vi "GDSProject_CreateFolder.vi"(0 "Project Refnum In":refnum<vi>, 1 "Project Item To Create Folder Below(Use MyComputer if not wired)":refnum<vi>, 3 "FolderName":string, 5 "error in (no error)":errorcluster, 7 "FolderScope":T1(array[ring]), 8 "CreateThePhysicalFolderIfPossible(False)":bool, 9 "GuessFolderScope(False)":bool) -> (14 "Project Refnum Out":refnum<vi>, 15 "ItemOut":refnum<vi>, 16 "FolderCreated":bool, 19 "error out":errorcluster)   [LabVIEW 2016]
panel:
  # "E.g. Private/SubPrivate"
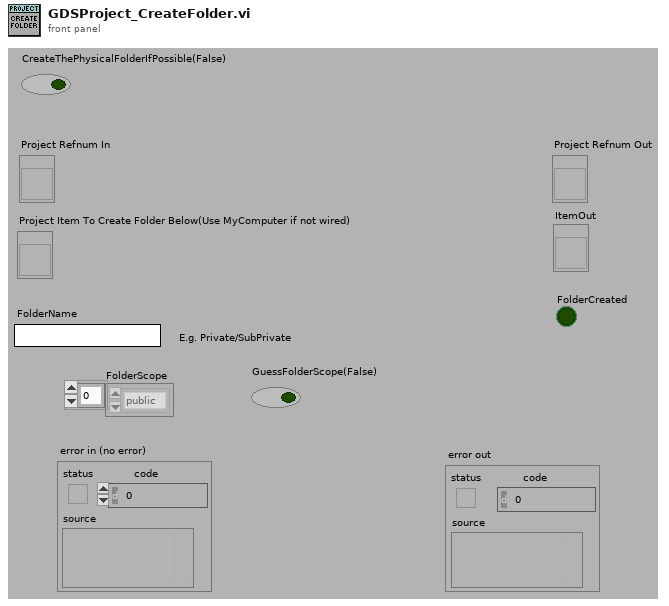
[diagram p1: front panel]
types:
  T1 = enum32{"invalid scope", "public", "private", "protected", "community"}[]
  T2 = enum32{"invalid scope", "public", "private", "protected"}
  T3 = enum32{"invalid scope", "public", "private", "protected", "community"}
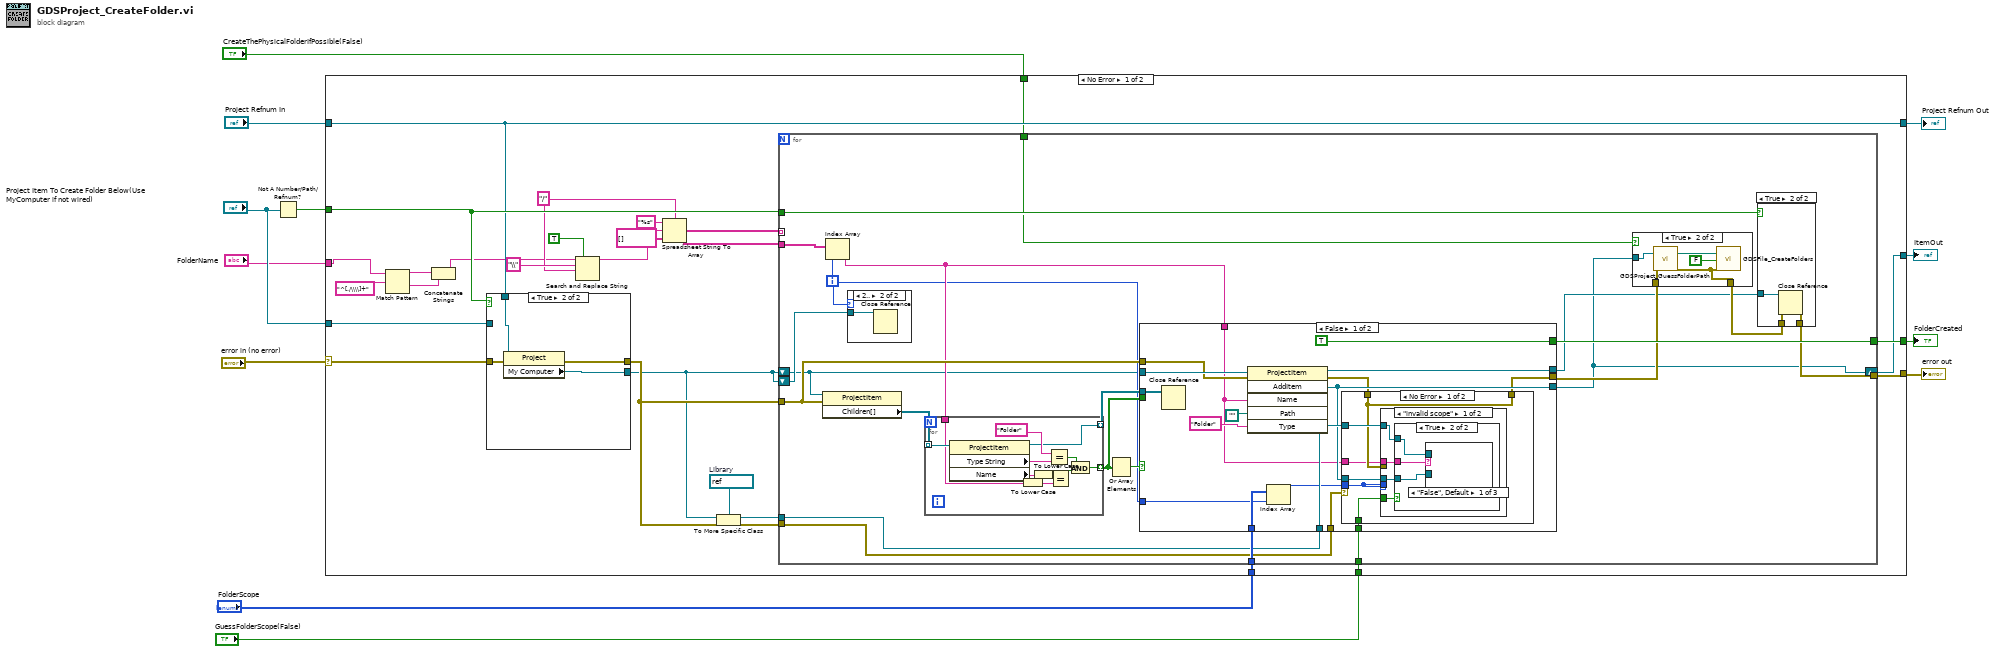
[diagram p0: block diagram]
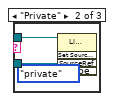
[diagram p5: hidden frame]
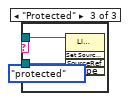
[diagram p6: hidden frame]
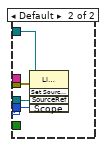
[diagram p7: hidden frame]
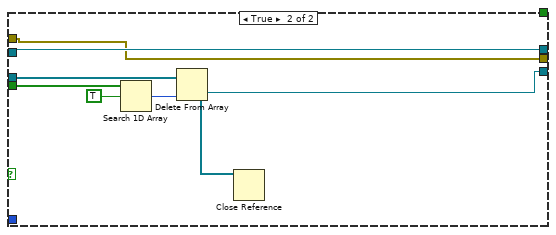
[diagram p9: hidden frame]
diagram:
  n1 = Not A Number/Path/Refnum?(number/path/refnum="Project Item To Create Folder Below(Use MyComputer if not wired)") -> (NaN/Path/Refnum?=w9:bool)
  n2 = case shown="No Error" "error in (no error)" {
    selector: "error in (no error)" -> [w39 w140]
    tunnel: [w33 w140] -> w11
    tunnel: "Project Refnum In" -> [w36 w139]
    tunnel: w9 -> [w37 _]
    tunnel: "Project Item To Create Folder Below(Use MyComputer if not wired)" -> [w38 _]
    tunnel: [w36 w139] -> w7
    tunnel: "FolderName" -> [w14 _]
    tunnel: [w29 _] -> w5
    tunnel: [w35 _] -> w4
    tunnel: "CreateThePhysicalFolderIfPossible(False)" -> [w34 _]
    tunnel: "FolderScope" -> [w28 _]
    tunnel: "GuessFolderScope(False)" -> [w18 _]
    frame No Error {
      w23 = refnum<vi> refnum  # Library
      w26 = "/" ("delimiter (Tab)")
      n3 = Match Pattern(string=w14, regular expression="^[./\\\\]+") -> (before substring=w16:string, after substring=w15:string)  [unwired: 1 in, 2 out]
      n4 = Concatenate Strings(w16, w15) -> (w13:string)
      n5 = case shown="True" w37 {
        tunnel: w36 -> [_ w138]
        tunnel: w39 -> [w133 w137]
        tunnel: [w134 w136] -> w19
        tunnel: w38 -> [w134 _]
        tunnel: [w133 w135] -> w20
        frame False {
        }
        frame True {
          n6 = property class="Project"(reference=w138, error in=w137) -> (error out=w135:errorcluster, "My Computer"=w136:refnum<vi>)  [unwired: 1 out]
        }
      }
      n7 = Search and Replace String(replace all?=TRUE ("replace all? (F)"), input string=w13, search string="\\", replace string=w26) -> (result string=w24:string)  [unwired: 4 in, 3 out]
      n8 = Spreadsheet String To Array(delimiter (Tab)=w26, format string="%s", spreadsheet string=w24, array type (2D Dbl)=string[] []) -> (array=w30:string[])
      n9 = To More Specific Class(target class=w23, reference=w19, error in=w20) -> (specific class reference=w22:refnum<vi>, error out=w21:errorcluster)
      n10 = for {
        tunnel: w37 -> [w61]
        tunnel: w20 -> [w60]
        tunnel: [w55] -> w35
        tunnel: w34 -> [w54]
        tunnel: [w51] -> w33
        tunnel: w30 -> [_] mode=indexing
        tunnel: w30 -> [w49]
        shift-right: [w47] -> w29
        shift-left: w19 -> [w43]
        shift-left: w19 -> [w46]
        tunnel: w28 -> [w45]
        tunnel: w22 -> [w42]
        tunnel: w21 -> [w41]
        tunnel: w18 -> [w40]
        i -> [w44]
        n11 = property class="ProjectItem"(reference=w43, error in=w60) -> ("Children[]"=w59:refnum<vi>[])  [unwired: 2 out]
        n12 = Index Array(array=w49, index=w44) -> (element=w48:string)
        n13 = case shown="2.." w44 {
          tunnel: w46 -> [_ w62]
          frame 0, Default {
          }
          frame 2.. {
            n14 = Close Reference(reference=w62) -> ()  [unwired: 1 in, 1 out]
          }
        }
        n15 = for {
          tunnel: w59 -> [w128] mode=indexing
          tunnel: w48 -> [w124]
          tunnel: [w121] -> w57 mode=indexing
          tunnel: [w120] -> w56 mode=indexing
          n16 = property class="ProjectItem"(reference=w128) -> (reference out=w120:refnum<vi>, "Type String"=w127:string, "Name"=w125:string)  [unwired: 1 in, 1 out]
          n17 = To Lower Case(string=w124) -> (all lower case string=w118:string)
          n18 = To Lower Case(string=w125) -> (all lower case string=w119:string)
          n19 = Equal?(x="Folder", y=w127) -> (x = y?=w123:bool)
          n20 = Equal?(x=w119, y=w118) -> (x = y?=w122:bool)
          n21 = And(x=w123, y=w122) -> (x .and. y?=w121:bool)
        }
        n22 = Or Array Elements(Boolean array=w57) -> (logical OR=w58:bool)
        n23 = case shown="False" w58 {
          tunnel: [w72 w111] -> w53
          tunnel: [w75 w113] -> w47
          tunnel: [w84 w112] -> w50
          tunnel: w43 -> [w82 w112]
          tunnel: w60 -> [w81 w111]
          tunnel: w48 -> [w70 _]
          tunnel: w57 -> [_ w117]
          tunnel: w56 -> [w69 w115]
          tunnel: [TRUE _] -> w55
          tunnel: w45 -> [w79 _]
          tunnel: w44 -> [w78 _]
          tunnel: w41 -> [w77 _]
          tunnel: w42 -> [w76 _]
          tunnel: w40 -> [w71 _]
          frame False {
            n24 = Close Reference(reference=w69) -> ()  [unwired: 1 in, 1 out]
            n25 = invoke class="ProjectItem" method="AddItem"(reference=w82, error in=w81, "Name"=w70, "Path"=path "", "Type"="Folder") -> (reference out=w84:refnum<vi>, error out=w73:errorcluster, "AddItem"=w75:refnum<vi>)  [unwired: 1 in, 3 out]
            n26 = Index Array(array=w79, index=w78) -> (element=w74:T3)
            n27 = case shown="No Error" w77 {
              tunnel: w76 -> [w91 _]
              tunnel: w75 -> [w90 _]
              tunnel: w74 -> [w89 _]
              tunnel: w73 -> [w88 w109]
              tunnel: [w88 w109] -> w72
              tunnel: w71 -> [w87 _]
              tunnel: w70 -> [w86 _]
              frame No Error {
                n28 = case shown="\"invalid scope\"" w89 {
                  tunnel: w91 -> [w93 w108]
                  tunnel: w90 -> [w94 w107]
                  tunnel: w88 -> [_ w106]
                  tunnel: w89 -> [_ w105]
                  tunnel: w87 -> [w95 _]
                  tunnel: w86 -> [w92 _]
                  frame "invalid scope" {
                    n29 = case shown="True" w95 {
                      tunnel: w94 -> [_ w97]
                      tunnel: w93 -> [_ w98]
                      tunnel: w92 -> [_ w96]
                      frame False {
                      }
                      frame True {
                        n30 = case shown="\"False\", Default" w96 {
                          tunnel: w98 -> [_ w101 w104]
                          tunnel: w97 -> [_ w100 w103]
                          frame "False", Default {
                          }
                          frame "Private" {
                            n31 = invoke class="Library" method="Set Source Scope"(reference=w101, "SourceRef"=w100, "Scope"=T2."private" ("scope")) -> ()  [unwired: 2 in, 5 out]
                          }
                          frame "Protected" {
                            n32 = invoke class="Library" method="Set Source Scope"(reference=w104, "SourceRef"=w103, "Scope"=T2."protected" ("scope")) -> ()  [unwired: 2 in, 5 out]
                          }
                        }
                      }
                    }
                  }
                  frame Default {
                    n33 = invoke class="Library" method="Set Source Scope"(reference=w108, error in=w106, "SourceRef"=w107, "Scope"=w105) -> ()  [unwired: 1 in, 5 out]
                  }
                }
              }
              frame Error {
              }
            }
          }
          frame True {
            n34 = Search 1D Array(1D array=w117, element=TRUE) -> (index of element=w114:i32)  [unwired: 1 in]
            n35 = Delete From Array(array=w115, index=w114) -> (deleted portion=w113:refnum<vi>, array with subset deleted=w110:refnum<vi>[])  [unwired: 1 in]
            n36 = Close Reference(reference=w110) -> ()  [unwired: 1 in, 1 out]
          }
        }
        n37 = case shown="True" w54 {
          tunnel: w53 -> [w63 w67]
          tunnel: [w63 w66] -> w52
          tunnel: w47 -> [_ w64]
          frame False {
          }
          frame True {
            n38 = call <resource>:"GDSProject_GuessFolderPath.vi"("ProjectItem"=w64, "error in (no error)"=w67) -> ("Path"=w68:path, "error out"=w66:errorcluster)  [unwired: 14 in, 2 out]
            n39 = call <resource>:"GDSFile_CreateFolders.vi"("Path"=w68, "Promt if folder\ndoes not exists?"=FALSE ("Promt if folder\ndoes not exists?"), "error in (no error)"=w66) -> ()  [unwired: 12 in, 5 out]
          }
        }
        n40 = case shown="True" w61 {
          tunnel: [w129 w132] -> w51
          tunnel: w50 -> [_ w131]
          tunnel: w52 -> [w129 w130]
          frame False {
          }
          frame True {
            n41 = Close Reference(reference=w131, error in (no error)=w130) -> (error out=w132:errorcluster)
          }
        }
      }
    }
    frame Error {
    }
  }
  "Project Refnum Out" <- w7
  "error out" <- w11
  "ItemOut" <- w5
  "FolderCreated" <- w4
